vi "Avg Dist To Left Wall (SubVI).vi"   [LabVIEW 2017]
uses:
  <vilib>/Analysis/baseanly.llb/Mean (DBL).vi
  <vilib>/Analysis/NI_AALBase.lvlib
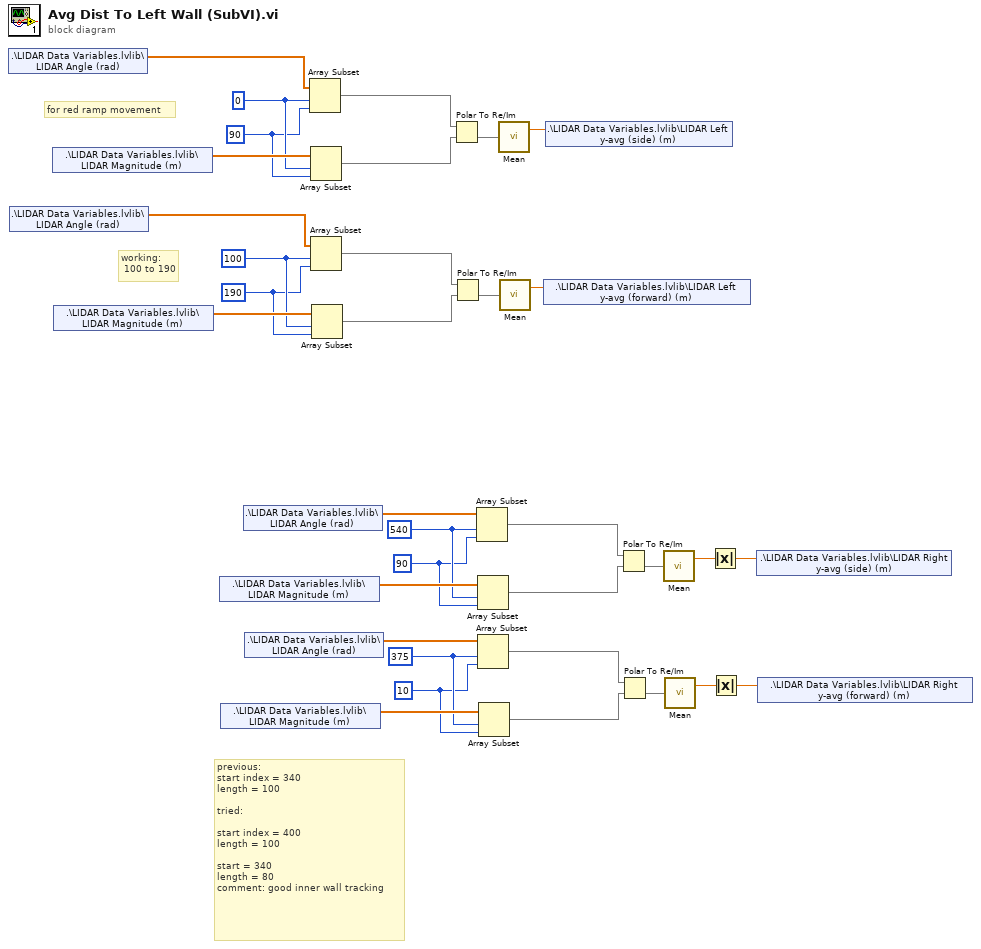
[diagram p0: block diagram]
diagram:
  w6 = 90 ("length")
  w7 = 540 ("index")
  w15 = 90 ("length")
  w16 = 0 ("index")
  w25 = 10 ("length")
  w26 = 375 ("index")
  w32 = 190 ("length")
  w33 = 100 ("index")
  # "previous:\nstart index = 340\nlength = 100\n\ntried:\n\nstart index = 400\nlength = 100\n\nstart = 340\nlength = 80\ncomment: good inner wall tracking"
  # "for red ramp movement"
  # "working:\n 100 to 190"
  n1 = shared-variable ".\\LIDAR Data Variables.lvlib\\LIDAR Angle (rad)"() -> (w12:dbl[])  [unwired: 1 in, 1 out]
  n2 = shared-variable ".\\LIDAR Data Variables.lvlib\\LIDAR Angle (rad)"() -> (w19:dbl[])  [unwired: 1 in, 1 out]
  n3 = shared-variable ".\\LIDAR Data Variables.lvlib\\LIDAR Magnitude (m)"() -> (w17:dbl[])  [unwired: 1 in, 1 out]
  n4 = shared-variable ".\\LIDAR Data Variables.lvlib\\LIDAR Magnitude (m)"() -> (w34:dbl[])  [unwired: 1 in, 1 out]
  n5 = shared-variable ".\\LIDAR Data Variables.lvlib\\LIDAR Magnitude (m)"() -> (w8:dbl[])  [unwired: 1 in, 1 out]
  n6 = shared-variable ".\\LIDAR Data Variables.lvlib\\LIDAR Magnitude (m)"() -> (w27:dbl[])  [unwired: 1 in, 1 out]
  n7 = shared-variable ".\\LIDAR Data Variables.lvlib\\LIDAR Angle (rad)"() -> (w9:dbl[])  [unwired: 1 in, 1 out]
  n8 = shared-variable ".\\LIDAR Data Variables.lvlib\\LIDAR Angle (rad)"() -> (w28:dbl[])  [unwired: 1 in, 1 out]
  n9 = Array Subset(array=w12, index=w16, length=w15) -> (w14:dbl[])
  n10 = Array Subset(array=w17, index=w16, length=w15) -> (w13:dbl[])
  n11 = Array Subset(array=w19, index=w33, length=w32) -> (w31:dbl[])
  n12 = Array Subset(array=w34, index=w33, length=w32) -> (w30:dbl[])
  n13 = Polar To Re/Im(2:w13, 3:w14) -> (0:w11:dbl[])  [unwired: 1 out]
  n14 = Polar To Re/Im(2:w30, 3:w31) -> (0:w18:dbl[])  [unwired: 1 out]
  n15 = Array Subset(array=w9, index=w7, length=w6) -> (w5:dbl[])
  n16 = Array Subset(array=w8, index=w7, length=w6) -> (w4:dbl[])
  n17 = Array Subset(array=w28, index=w26, length=w25) -> (w24:dbl[])
  n18 = Array Subset(array=w27, index=w26, length=w25) -> (w23:dbl[])
  n19 = call-poly <vilib>:"Mean.vi"("X"=w11) -> ("mean"=w10:dbl)  [unwired: 1 out]
  n20 = call-poly <vilib>:"Mean.vi"("X"=w18) -> ("mean"=w29:dbl)  [unwired: 1 out]
  n21 = shared-variable ".\\LIDAR Data Variables.lvlib\\LIDAR Left y-avg (forward) (m)"(w29) -> ()  [unwired: 1 in, 1 out]
  n22 = shared-variable ".\\LIDAR Data Variables.lvlib\\LIDAR Left y-avg (side) (m)"(w10) -> ()  [unwired: 1 in, 1 out]
  n23 = Polar To Re/Im(2:w4, 3:w5) -> (0:w3:dbl[])  [unwired: 1 out]
  n24 = Polar To Re/Im(2:w23, 3:w24) -> (0:w22:dbl[])  [unwired: 1 out]
  n25 = call-poly <vilib>:"Mean.vi"("X"=w3) -> ("mean"=w2:dbl)  [unwired: 1 out]
  n26 = call-poly <vilib>:"Mean.vi"("X"=w22) -> ("mean"=w21:dbl)  [unwired: 1 out]
  n27 = Absolute Value(x=w2) -> (abs(x)=w1:dbl)
  n28 = Absolute Value(x=w21) -> (abs(x)=w20:dbl)
  n29 = shared-variable ".\\LIDAR Data Variables.lvlib\\LIDAR Right y-avg (side) (m)"(w1) -> ()  [unwired: 1 in, 1 out]
  n30 = shared-variable ".\\LIDAR Data Variables.lvlib\\LIDAR Right y-avg (forward) (m)"(w20) -> ()  [unwired: 1 in, 1 out]
